vi "INTERFACE_HW_SW_FUERZA_PRENSIL_2009.vi"() -> ()   [LabVIEW 2009]
uses:
  <vilib>/Instr/_visa.llb/VISA Set IO Buffer Mask.ctl
  <vilib>/Instr/_visa.llb/VISA Configure Serial Port (Instr).vi
panel:
  out "GRAFICA DE LA FUERZA PRENSIL":cluster{dbl[], dbl[]}[](graph)
  out "F1":dbl format="%#_2g"
  out "F2":dbl format="%#_2g"
  out "F3":dbl format="%#_2g"
  in  "stop":bool
  out "Slide":u16(slide) scale=0.0..15.0
  out "Slide 2":u16(slide) scale=0.0..15.0
  out "Slide 3":u16(slide) scale=0.0..15.0
  out "Slide 4":u16(slide) scale=0.0..15.0
  out "Fprom":dbl format="%#_2g"
  out "F1 media":dbl format="%#.2g"
  out "F1 Max":dbl format="%#.2g"
  out "F2 media":dbl format="%#.2g"
  out "F2 Max":dbl format="%#.2g"
  out "F3 media":dbl format="%#.2g"
  out "F3 Max":dbl format="%#.2g"
  out "Fprom media":dbl format="%#.2g"
  out "Fprom Max":dbl format="%#.2g"
  out "Slide 5":u16(slide) scale=0.0..15.0 scale format="%.2f"
  out "F4":dbl format="%#_2g"
  out "F4 Max":dbl format="%#_2g"
  out "F4 Media":dbl format="%#_2g"
  out "No. de muestra":i32
  in  "MEDIR":bool
  out "Fprensil (N)":dbl
  out "Fprensil (kgf)":dbl
  in  "VISA resource name":refnum<visa-resource-name>
  # "L"
  # "i"
  # "V"
  # "INTERFASE PARA LA MEDICIÓN DE LA FUERZA PRENSIL"
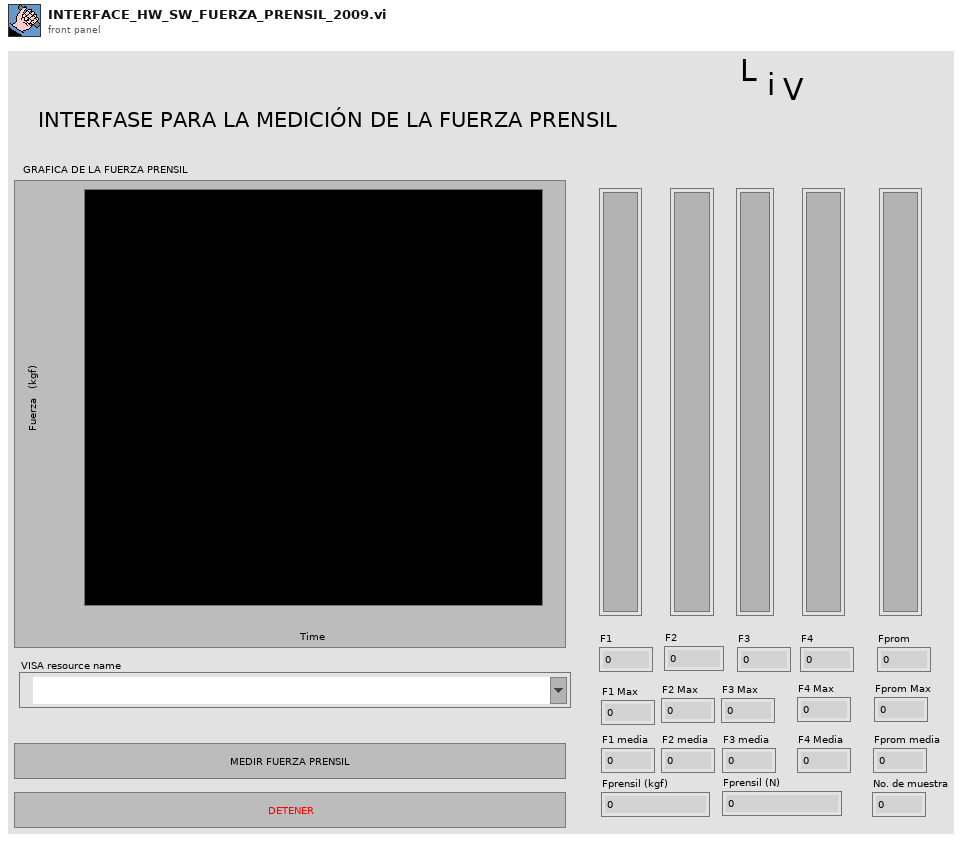
[diagram p1: front panel]
types:
  T1 = typedef "VISA Set IO Buffer Mask.ctl" = u16
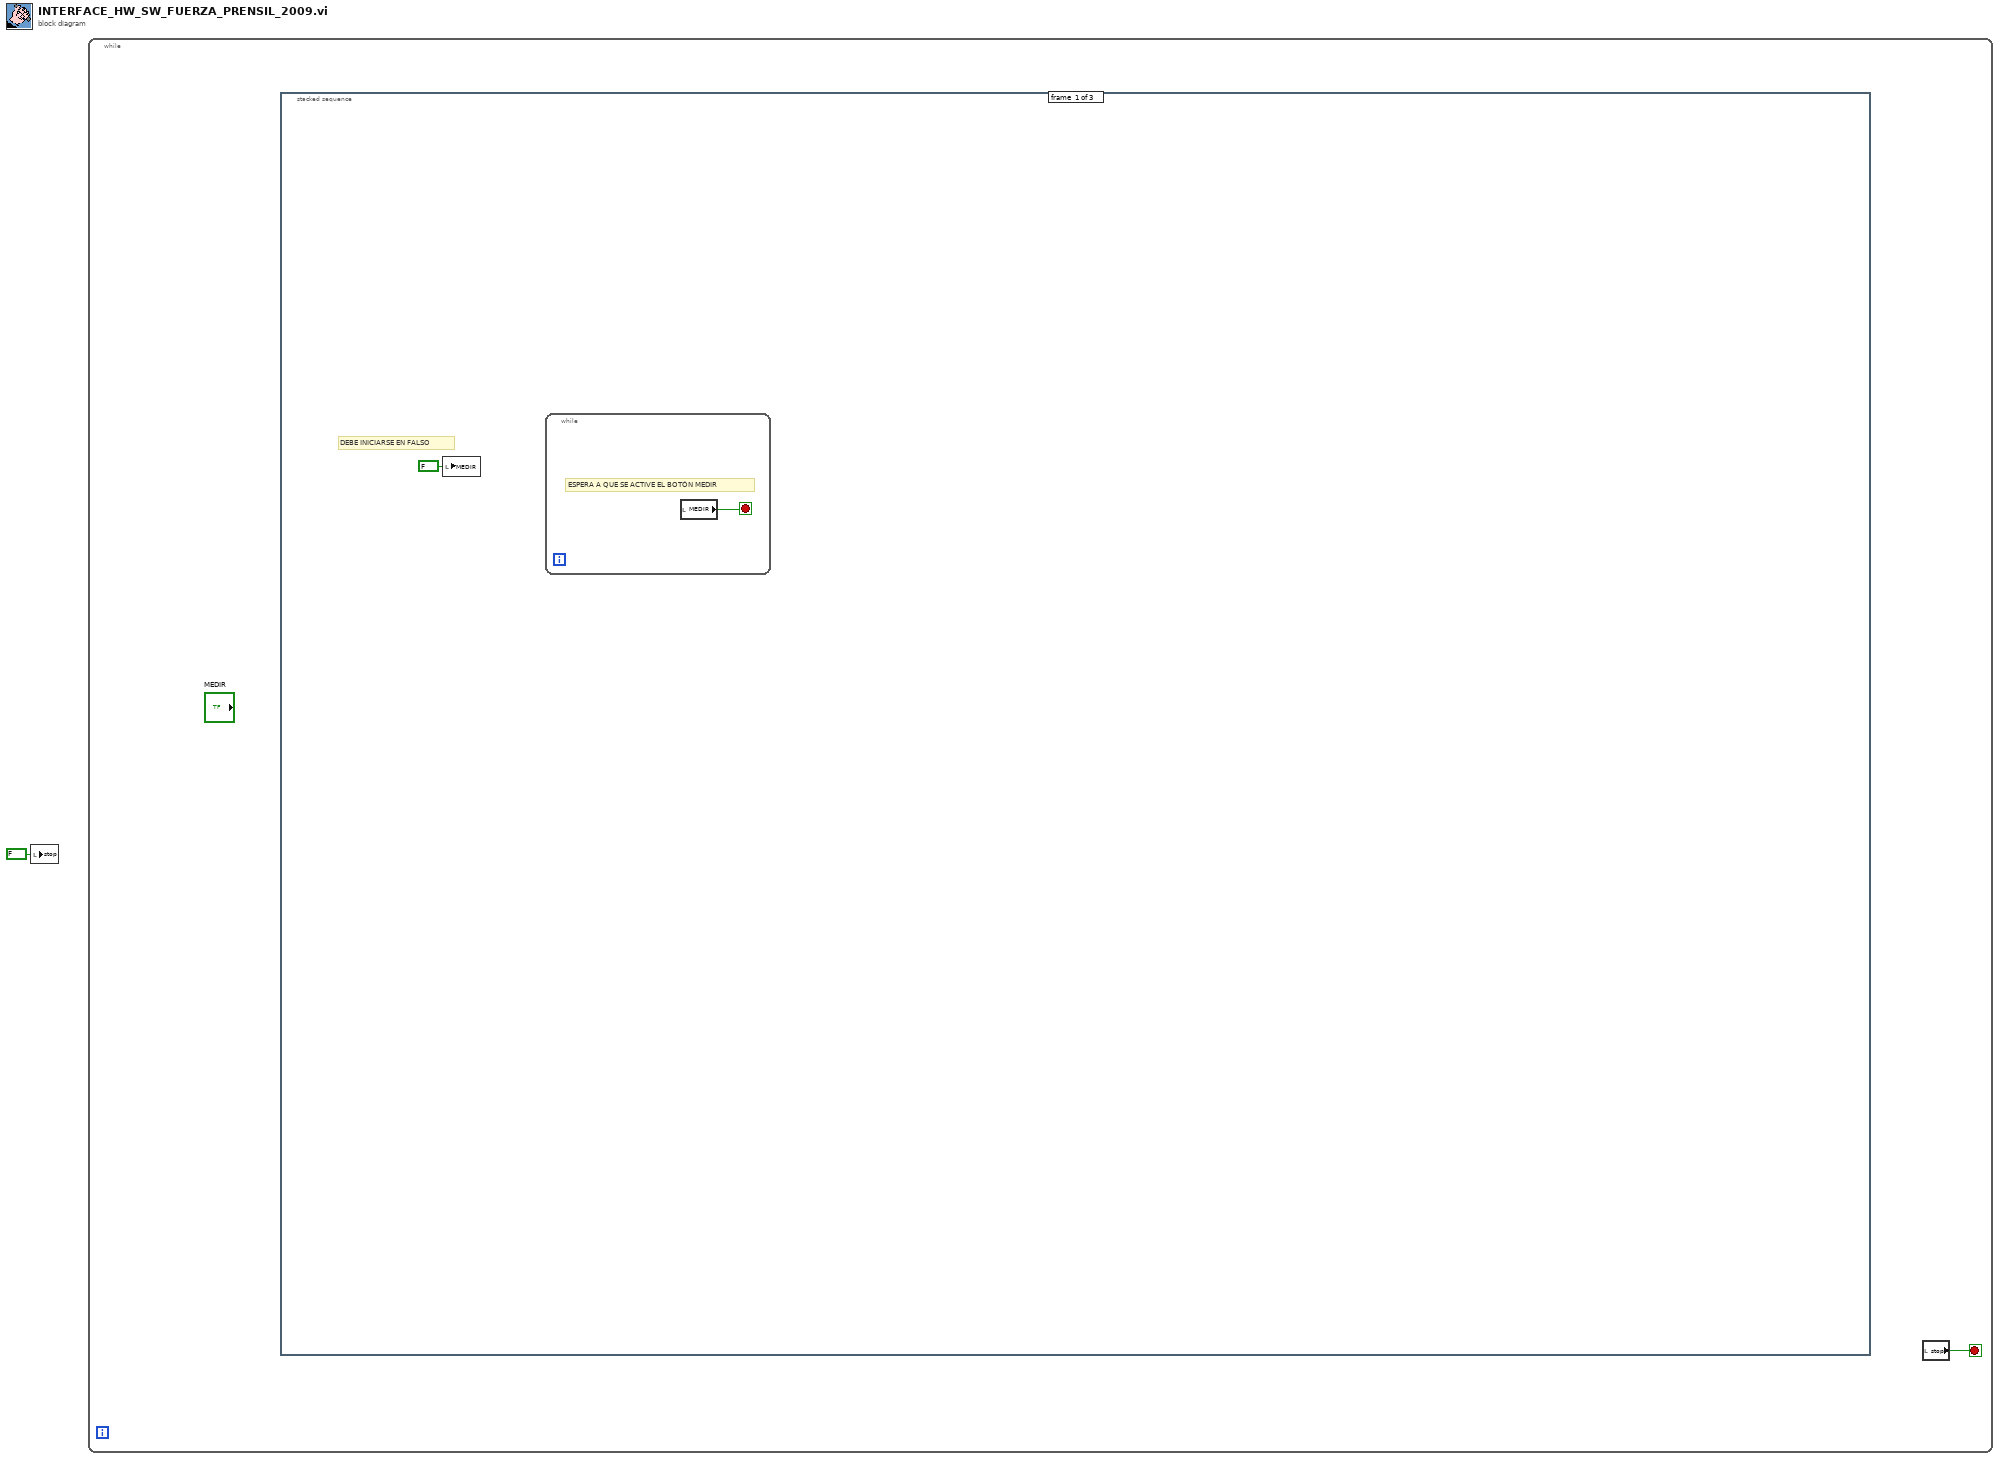
[diagram p0: block diagram]
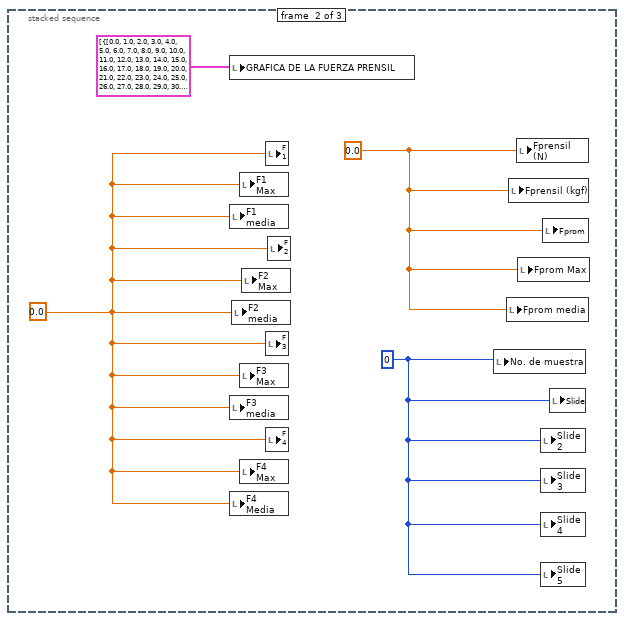
[diagram p2: hidden frame]
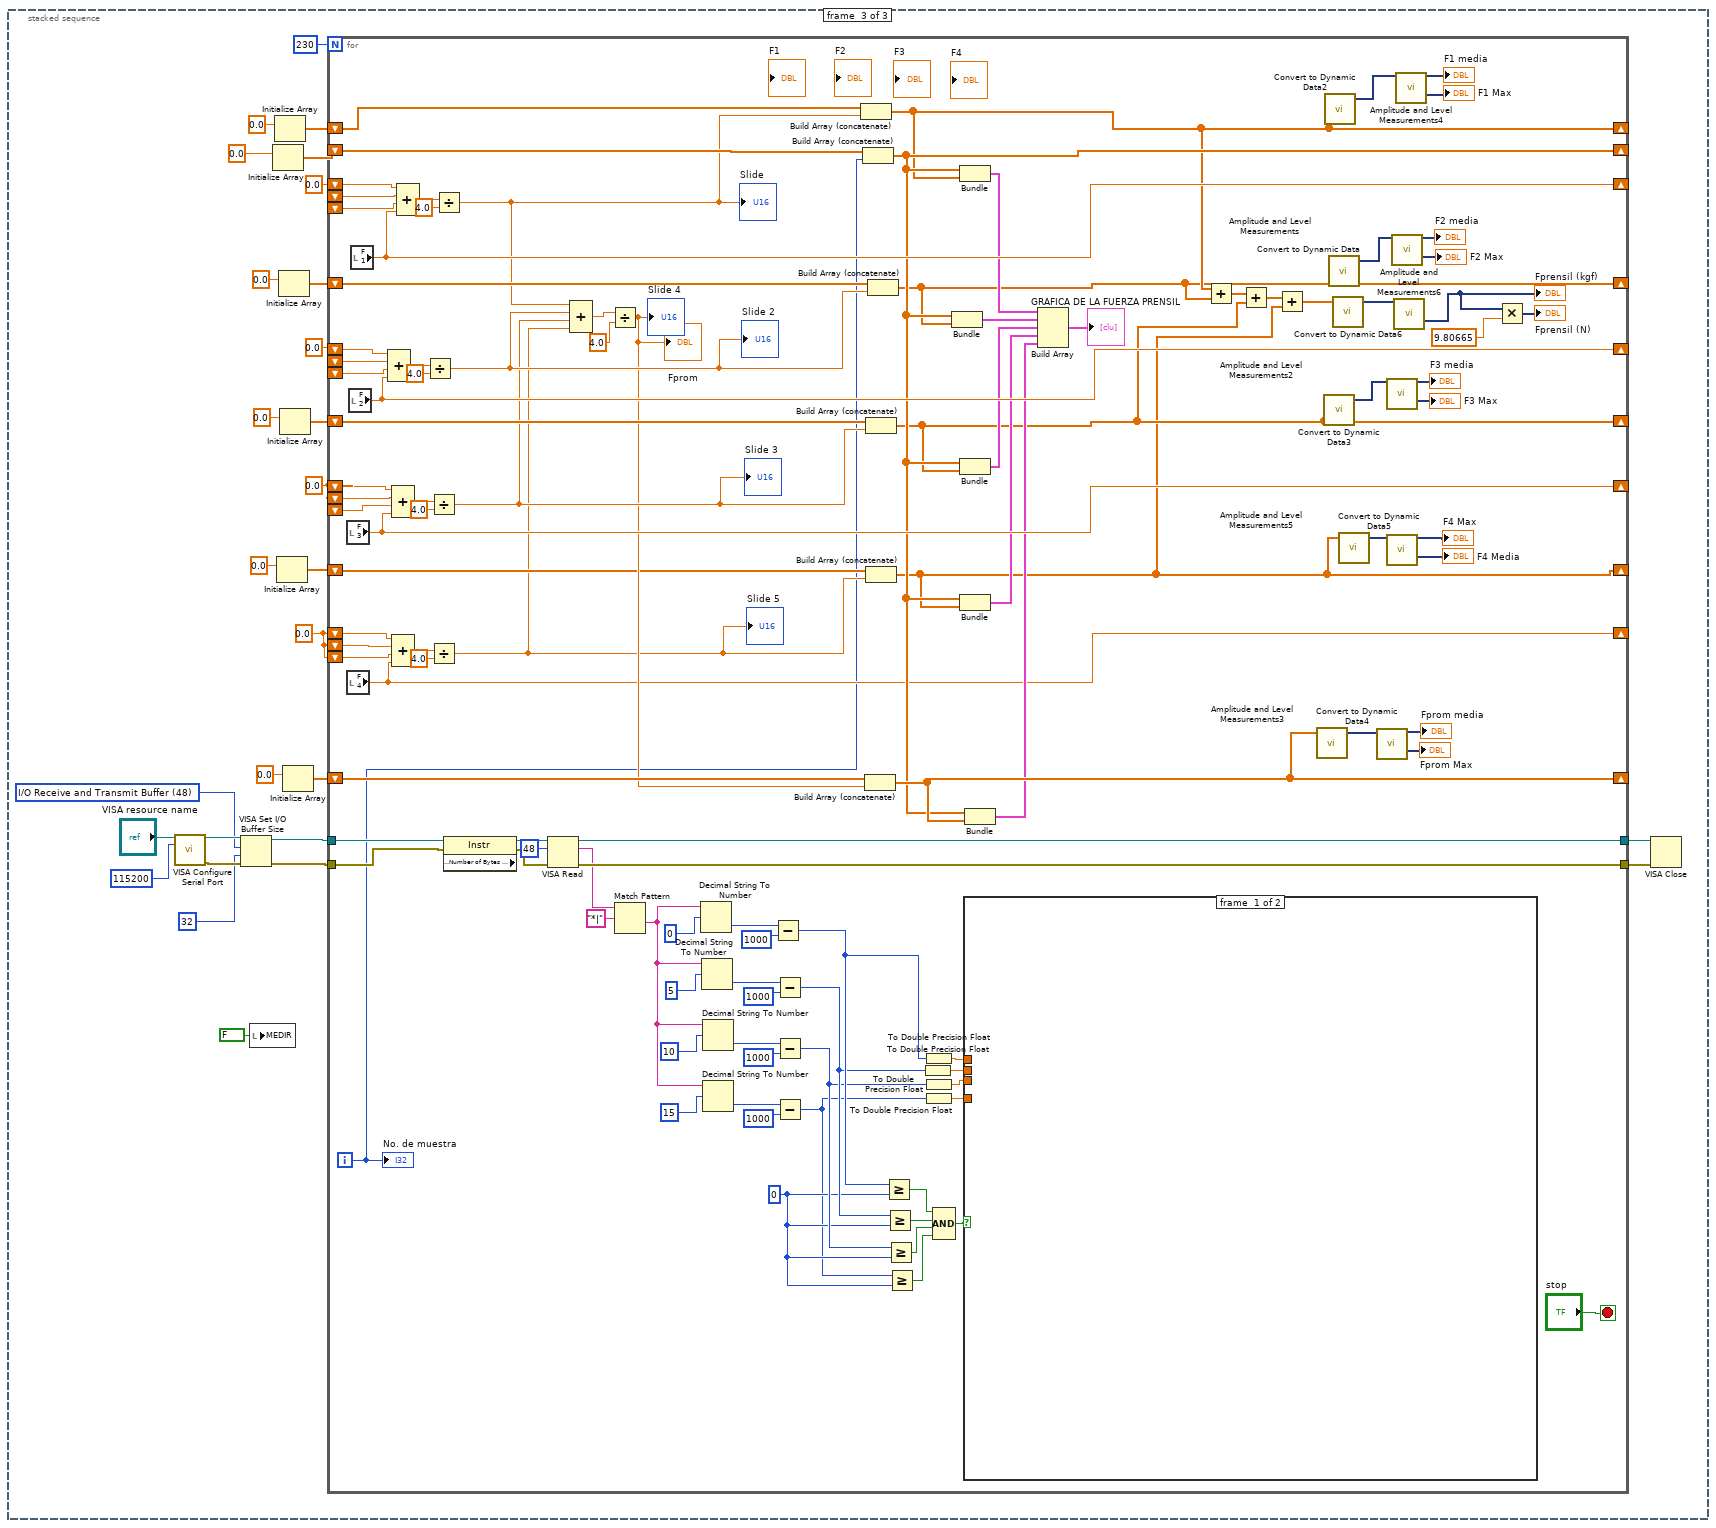
[diagram p3: hidden frame]
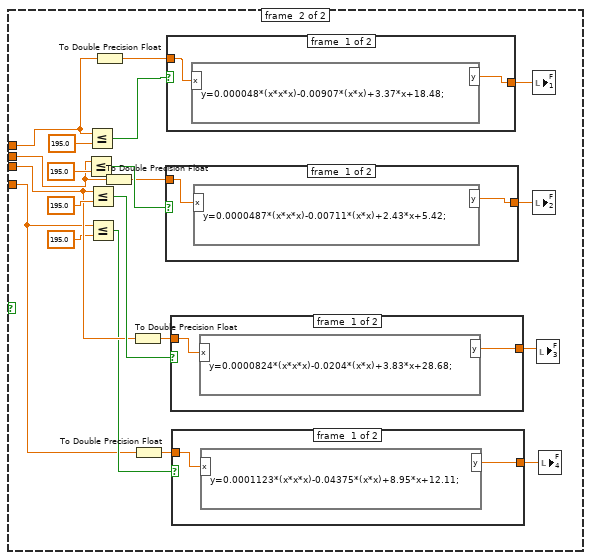
[diagram p4: hidden frame]
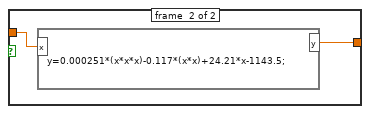
[diagram p5: hidden frame]
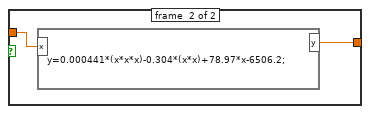
[diagram p6: hidden frame]
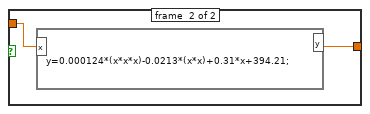
[diagram p7: hidden frame]
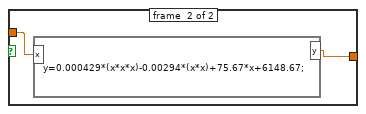
[diagram p8: hidden frame]
diagram:
  n1 = local write "stop"(FALSE ("stop")) -> ()
  n2 = while {
    stop <- w2 stop-if-true
    n3 = stacked-sequence {
      frame #0 {
        # "DEBE INICIARSE EN FALSO"
        n4 = local write "MEDIR"(FALSE ("MEDIR")) -> ()
        n5 = while {
          stop <- w4 stop-if-true
          # "ESPERA A QUE SE ACTIVE EL BOTÓN MEDIR"
          n6 = local read "MEDIR"() -> (w4:bool)
        }
      }
      frame #1 {
        w5 = 0.0 ("Fprensil (N)")
        w6 = 0.0 ("F1")
        w7 = 0 ("No. de muestra")
        n7 = local write "GRAFICA DE LA FUERZA PRENSIL"(cluster{dbl[], dbl[]}[] [{[0.0, 1.0, 2.0, 3.0, 4.0, 5.0, 6.0, 7.0, 8.0, 9.0, 10.0, 11.0, 12.0, 13.0, 14.0, 15.0, 16.0, 17.0, 18.0, 19.0, 20.0, 21.0, 22.0, 23.0, 24.0, 25.0, 26.0, 27.0, 28.0, 29.0, 30.0, 31.0, 32.0, 33.0, 34.0, 35.0, 36.0, 37.0, 38.0, 39.0, 40.0, 41.0, 42.0, 43.0, 44.0, 45.0, 46.0, 47.0, 48.0, 49.0, 50.0, 51.0, 52.0, 53.0, 54.0, 55.0, 56.0, 57.0, 58.0, 59.0, 60.0, 61.0, 62.0, 63.0, 64.0, 65.0, 66.0, 67.0, 68.0, 69.0, 70.0, 71.0, 72.0, 73.0, 74.0, 75.0, 76.0, 77.0, 78.0, 79.0, 80.0, 81.0, 82.0, 83.0, 84.0, 85.0, 86.0, 87.0, 88.0, 89.0, 90.0, 91.0, 92.0, 93.0, 94.0, 95.0, 96.0, 97.0, 98.0, 99.0, 100.0, 101.0, 102.0, 103.0, 104.0, 105.0, 106.0, 107.0, 108.0, 109.0, 110.0, 111.0, 112.0, 113.0, 114.0, 115.0, 116.0, 117.0, 118.0, 119.0, 120.0, 121.0, 122.0, 123.0, 124.0, 125.0, 126.0, 127.0, 128.0, 129.0, 130.0, 131.0, 132.0, 133.0, 134.0, 135.0, 136.0, 137.0, 138.0, 139.0, 140.0, 141.0, 142.0, 143.0, 144.0, 145.0, 146.0, 147.0, 148.0, 149.0, 150.0, 151.0, 152.0, 153.0, 154.0, 155.0, 156.0, 157.0, 158.0, 159.0, 160.0, 161.0, 162.0, 163.0, 164.0, 165.0, 166.0, 167.0, 168.0, 169.0, 170.0, 171.0, 172.0, 173.0, 174.0, 175.0, 176.0, 177.0, 178.0, 179.0, 180.0, 181.0, 182.0, 183.0, 184.0, 185.0, 186.0, 187.0, 188.0, 189.0, 190.0, 191.0, 192.0, 193.0, 194.0, 195.0, 196.0, 197.0, 198.0, 199.0, 200.0, 201.0, 202.0, 203.0, 204.0, 205.0, 206.0, 207.0, 208.0, 209.0, 210.0, 211.0, 212.0, 213.0, 214.0, 215.0, 216.0, 217.0, 218.0, 219.0, 220.0, 221.0, 222.0, 223.0, 224.0, 225.0, 226.0, 227.0, 228.0, 229.0], [0.0006720016874999999, 0.0013440033749999999, 0.0020160050625, 0.0026880067499999998, 0.0026880067499999998, 0.0026880067499999998, 0.0026880067499999998, 0.0026880067499999998, 0.0026880067499999998, 0.0026880067499999998, 0.0026880067499999998, 0.0026880067499999998, 0.0026880067499999998, 0.0026880067499999998, 0.0026880067499999998, 0.0026880067499999998, 0.0026880067499999998, 0.0026880067499999998, 0.0026880067499999998, 0.0026880067499999998, 0.0026880067499999998, 0.0026880067499999998, 0.0026880067499999998, 0.0026880067499999998, 0.0026880067499999998, 0.0026880067499999998, 0.0026880067499999998, 0.0026880067499999998, 0.0026880067499999998, 0.0026880067499999998, 0.0026880067499999998, 0.0026880067499999998, 0.0026880067499999998, 0.0026880067499999998, 0.0026880067499999998, 0.0026880067499999998, 0.0026880067499999998, 0.0026880067499999998, 0.0026880067499999998, 0.0026880067499999998, 0.0026880067499999998, 0.0026880067499999998, 0.0026880067499999998, 0.0026880067499999998, 0.0026880067499999998, 0.0026880067499999998, 0.0026880067499999998, 0.0026880067499999998, 0.0026880067499999998, 0.0026880067499999998, 0.0026880067499999998, 0.0026880067499999998, 0.0026880067499999998, 0.0026880067499999998, 0.0026880067499999998, 0.0026880067499999998, 0.0026880067499999998, 0.0026880067499999998, 0.0026880067499999998, 0.0026880067499999998, 0.0026880067499999998, 0.0026880067499999998, 0.0026880067499999998, 0.0026880067499999998, 0.0026880067499999998, 0.0026880067499999998, 0.0026880067499999998, 0.0026880067499999998, 0.0026880067499999998, 0.0026880067499999998, 0.0026880067499999998, 0.0026880067499999998, 0.0026880067499999998, 0.0026880067499999998, 0.0026880067499999998, 0.0026880067499999998, 0.0026880067499999998, 0.0026880067499999998, 0.0026880067499999998, 0.0026880067499999998, 0.0026880067499999998, 0.0026880067499999998, 0.0026880067499999998, 0.0026880067499999998, 0.0026880067499999998, 0.0026880067499999998, 0.0026880067499999998, 0.0026880067499999998, 0.0026880067499999998, 0.0026880067499999998, 0.0026880067499999998, 0.0026880067499999998, 0.0026880067499999998, 0.0026880067499999998, 0.0026880067499999998, 0.0026880067499999998, 0.0026880067499999998, 0.0026880067499999998, 0.0026880067499999998, 0.0026880067499999998, 0.0026880067499999998, 0.0026880067499999998, 0.0026880067499999998, 0.0026880067499999998, 0.0026880067499999998, 0.0026880067499999998, 0.0026880067499999998, 0.0026880067499999998, 0.0026880067499999998, 0.0026880067499999998, 0.0026880067499999998, 0.0026880067499999998, 0.0026880067499999998, 0.0026880067499999998, 0.0026880067499999998, 0.0026880067499999998, 0.0026880067499999998, 0.0026880067499999998, 0.0026880067499999998, 0.0026880067499999998, 0.0026880067499999998, 0.0026880067499999998, 0.0026880067499999998, 0.0026880067499999998, 0.0026880067499999998, 0.0026880067499999998, 0.0026880067499999998, 0.0026880067499999998, 0.0026880067499999998, 0.0026880067499999998, 0.0026880067499999998, 0.0026880067499999998, 0.0026880067499999998, 0.0026880067499999998, 0.0026880067499999998, 0.0026880067499999998, 0.0026880067499999998, 0.0026880067499999998, 0.0026880067499999998, 0.0026880067499999998, 0.0026880067499999998, 0.0026880067499999998, 0.0026880067499999998, 0.0026880067499999998, 0.0026880067499999998, 0.0026880067499999998, 0.0026880067499999998, 0.0026880067499999998, 0.0026880067499999998, 0.0026880067499999998, 0.0026880067499999998, 0.0026880067499999998, 0.0026880067499999998, 0.0026880067499999998, 0.0026880067499999998, 0.0026880067499999998, 0.0026880067499999998, 0.0026880067499999998, 0.0026880067499999998, 0.0026880067499999998, 0.0026880067499999998, 0.0026880067499999998, 0.0026880067499999998, 0.0026880067499999998, 0.0026880067499999998, 0.0026880067499999998, 0.0026880067499999998, 0.0026880067499999998, 0.0026880067499999998, 0.0026880067499999998, 0.0026880067499999998, 0.0026880067499999998, 0.0026880067499999998, 0.0026880067499999998, 0.0026880067499999998, 0.0026880067499999998, 0.0026880067499999998, 0.0026880067499999998, 0.0026880067499999998, 0.0026880067499999998, 0.0026880067499999998, 0.0026880067499999998, 0.0026880067499999998, 0.0026880067499999998, 0.0026880067499999998, 0.0026880067499999998, 0.0026880067499999998, 0.0026880067499999998, 0.0026880067499999998, 0.0026880067499999998, 0.0026880067499999998, 0.0026880067499999998, 0.0026880067499999998, 0.0026880067499999998, 0.0026880067499999998, 0.0026880067499999998, 0.0026880067499999998, 0.0026880067499999998, 0.0026880067499999998, 0.0026880067499999998, 0.0026880067499999998, 0.0026880067499999998, 0.0026880067499999998, 0.0026880067499999998, 0.0026880067499999998, 0.0026880067499999998, 0.0026880067499999998, 0.0026880067499999998, 0.0026880067499999998, 0.0026880067499999998, 0.0026880067499999998, 0.0026880067499999998, 0.0026880067499999998, 0.0026880067499999998, 0.0026880067499999998, 0.0026880067499999998, 0.0026880067499999998, 0.0026880067499999998, 0.0026880067499999998, 0.0026880067499999998, 0.0026880067499999998, 0.0026880067499999998, 0.0026880067499999998, 0.0026880067499999998, 0.0026880067499999998, 0.0026880067499999998, 0.0026880067499999998, 0.0026880067499999998, 0.0026880067499999998, 0.0026880067499999998]}, ...(5 in all)] ("GRAFICA DE LA FUERZA PRENSIL")) -> ()
        n8 = local write "F1 media"(w6) -> ()
        n9 = local write "F3 media"(w6) -> ()
        n10 = local write "F4 Media"(w6) -> ()
        n11 = local write "F2 media"(w6) -> ()
        n12 = local write "F1 Max"(w6) -> ()
        n13 = local write "F3 Max"(w6) -> ()
        n14 = local write "F4 Max"(w6) -> ()
        n15 = local write "F2 Max"(w6) -> ()
        n16 = local write "F1"(w6) -> ()
        n17 = local write "F3"(w6) -> ()
        n18 = local write "F4"(w6) -> ()
        n19 = local write "F2"(w6) -> ()
        n20 = local write "No. de muestra"(w7) -> ()
        n21 = local write "Fprom media"(w5) -> ()
        n22 = local write "Fprensil (kgf)"(w5) -> ()
        n23 = local write "Fprensil (N)"(w5) -> ()
        n24 = local write "Fprom Max"(w5) -> ()
        n25 = local write "Slide 2"(w7) -> ()
        n26 = local write "Slide 3"(w7) -> ()
        n27 = local write "Slide 4"(w7) -> ()
        n28 = local write "Slide 5"(w7) -> ()
        n29 = local write "Fprom"(w5) -> ()
        n30 = local write "Slide"(w7) -> ()
      }
      frame #2 {
        w14 = T1 48 items=["I/O Receive Buffer"=16, "I/O Transmit Buffer"=32, "I/O Receive and Transmit Buffer"=48] ("Mask")
        w20 = 0.0
        w29 = 0.0
        w30 = 0.0
        w34 = 0.0
        n31 = call-poly "VISA Configure Serial Port"("VISA resource name"="VISA resource name", "baud rate (9600)"=u32 115200) -> ("VISA resource name out"=w17:refnum<visa-resource-name>, "error out"=w18:errorcluster)  [unwired: 12 in]
        n32 = VISA Set I/O Buffer Size(VISA resource name=w17, mask (16)=w14, size (4096)=u32 32, error in (no error)=w18) -> (VISA resource name out=w12:refnum<visa-resource-name>, error out=w11:errorcluster)
        n33 = local write "MEDIR"(FALSE ("MEDIR")) -> ()
        n34 = Initialize Array(0.0 ("element")) -> (w31:dbl[])  [unwired: 1 in]
        n35 = Initialize Array(0.0 ("element")) -> (w32:dbl[])  [unwired: 1 in]
        n36 = Initialize Array(0.0 ("element")) -> (w21:dbl[])  [unwired: 1 in]
        n37 = Initialize Array(0.0 ("element")) -> (w26:dbl[])  [unwired: 1 in]
        n38 = Initialize Array(0.0 ("element")) -> (w25:dbl[])  [unwired: 1 in]
        n39 = Initialize Array(0.0 ("element")) -> (w23:dbl[])  [unwired: 1 in]
        n40 = for {
          N: 230 -> [_]
          tunnel: [w142] -> w10
          tunnel: [w141] -> w9
          tunnel: w12 -> [w130]
          tunnel: w11 -> [w129]
          shift-right: [w105] -> _
          shift-left: w34 -> [w124]
          shift-left: w34 -> [w123]
          shift-left: w34 -> [w122]
          shift-right: [w45] -> _
          shift-left: w32 -> [w119]
          shift-right: [w64] -> _
          shift-left: w31 -> [w118]
          shift-right: [w104] -> _
          shift-left: w30 -> [w115]
          shift-left: w30 -> [w114]
          shift-left: w30 -> [w113]
          shift-right: [w103] -> _
          shift-left: w29 -> [w110]
          shift-left: w29 -> [w109]
          shift-left: w29 -> [w108]
          shift-right: [w44] -> _
          shift-left: w26 -> [w107]
          shift-right: [w43] -> _
          shift-left: w25 -> [w106]
          shift-right: [w80] -> _
          shift-left: w23 -> [w91]
          shift-right: [w42] -> _
          shift-left: w21 -> [w70]
          shift-right: [w59] -> _
          shift-left: w20 -> [w67]
          shift-left: w20 -> [w66]
          shift-left: w20 -> [w65]
          i -> [w49]
          stop <- "stop" stop-if-true
          w56 = 0 ("y")
          n41 = local read "F3"() -> (w103:dbl)
          n42 = local read "F4"() -> (w59:dbl)
          n43 = local read "F2"() -> (w104:dbl)
          n44 = local read "F1"() -> (w105:dbl)
          n45 = Compound Arithmetic op=ADD(w115, w114, w113, w104) -> (w117:dbl)
          n46 = Compound Arithmetic op=ADD(w110, w109, w108, w103) -> (w112:dbl)
          n47 = Compound Arithmetic op=ADD(w67, w66, w65, w59) -> (w69:dbl)
          n48 = Compound Arithmetic op=ADD(w124, w123, w122, w105) -> (w121:dbl)
          n49 = Divide(x=w117, y=4.0) -> (x/y=w95:dbl)
          "Slide 2" <- w95
          n50 = Divide(x=w112, y=4.0) -> (x/y=w94:dbl)
          "Slide 3" <- w94
          n51 = Divide(x=w69, y=4.0) -> (x/y=w51:dbl)
          "Slide 5" <- w51
          n52 = Divide(x=w121, y=4.0) -> (x/y=w96:dbl)
          "Slide" <- w96
          n53 = property class="Instr" props=["Serial Settings:Number of Bytes at Serial Port"](reference=w130, error in=w129) -> (reference out=w145:refnum<visa-resource-name>, error out=w144:errorcluster)  [unwired: 1 out]
          n54 = VISA Read(VISA resource name=w145, byte count=u32 48, error in (no error)=w144) -> (VISA resource name out=w142:refnum<visa-resource-name>, read buffer=w131:string, error out=w141:errorcluster)  [unwired: 1 out]
          n55 = Compound Arithmetic op=ADD(w96, w95, w94, w51) -> (w93:dbl)
          n56 = Divide(x=w93, y=4.0) -> (x/y=w90:dbl)
          "Slide 4" <- w90
          "Fprom" <- w90
          n57 = Match Pattern(string=w131, regular expression="*|") -> (after substring=w52:string)  [unwired: 1 in, 3 out]
          n58 = Decimal String To Number(string=w52, offset=0) -> (number=w137:i32)  [unwired: 1 in, 1 out]
          n59 = Decimal String To Number(string=w52, offset=5) -> (number=w133:i32)  [unwired: 1 in, 1 out]
          n60 = Decimal String To Number(string=w52, offset=10) -> (number=w132:i32)  [unwired: 1 in, 1 out]
          n61 = Decimal String To Number(string=w52, offset=15) -> (number=w53:i32)  [unwired: 1 in, 1 out]
          n62 = Subtract(x=w137, y=1000) -> (x-y=w89:i32)
          n63 = Subtract(x=w133, y=1000) -> (x-y=w87:i32)
          n64 = Subtract(x=w132, y=1000) -> (x-y=w85:i32)
          n65 = Subtract(x=w53, y=1000) -> (x-y=w48:i32)
          n66 = Build Array (concatenate)(w119, w96) -> (w45:dbl[])
          n67 = Build Array (concatenate)(w118, w49) -> (w64:dbl[])
          n68 = Build Array (concatenate)(w91, w90) -> (w80:dbl[])
          n69 = Build Array (concatenate)(w106, w94) -> (w43:dbl[])
          n70 = Build Array (concatenate)(w70, w51) -> (w42:dbl[])
          n71 = Build Array (concatenate)(w107, w95) -> (w44:dbl[])
          n72 = Greater Or Equal?(x=w89, y=w56) -> (x >= y?=w127:bool)
          n73 = Greater Or Equal?(x=w87, y=w56) -> (x >= y?=w128:bool)
          n74 = Greater Or Equal?(x=w85, y=w56) -> (x >= y?=w126:bool)
          n75 = Greater Or Equal?(x=w48, y=w56) -> (x >= y?=w57:bool)
          n76 = To Double Precision Float(number=w87) -> (double precision float=w86:dbl)
          n77 = To Double Precision Float(number=w89) -> (double precision float=w88:dbl)
          n78 = To Double Precision Float(number=w85) -> (double precision float=w84:dbl)
          n79 = To Double Precision Float(number=w48) -> (double precision float=w58:dbl)
          n80 = Compound Arithmetic op=AND(w127, w128, w126, w57) -> (w125:bool)
          n81 = Bundle(w64, w44) -> (w101:cluster{dbl[], dbl[]})  [unwired: 1 in]
          n82 = Bundle(w64, w45) -> (w102:cluster{dbl[], dbl[]})  [unwired: 1 in]
          n83 = Bundle(w64, w43) -> (w100:cluster{dbl[], dbl[]})  [unwired: 1 in]
          n84 = Bundle(w64, w42) -> (w62:cluster{dbl[], dbl[]})  [unwired: 1 in]
          n85 = case shown="True" w125 {
            tunnel: w88 -> [_ w159]
            tunnel: w86 -> [_ w154]
            tunnel: w84 -> [_ w157]
            tunnel: w58 -> [_ w146]
            frame #0 {
            }
            frame #1 {
              n86 = Less Or Equal?(x=w154, y=195.0) -> (x <= y?=w161:bool)
              n87 = Less Or Equal?(x=w159, y=195.0) -> (x <= y?=w162:bool)
              n88 = Less Or Equal?(x=w157, y=195.0) -> (x <= y?=w160:bool)
              n89 = Less Or Equal?(x=w146, y=195.0) -> (x <= y?=w147:bool)
              n90 = To Double Precision Float(number=w159) -> (double precision float=w158:dbl)
              n91 = To Double Precision Float(number=w154) -> (double precision float=w155:dbl)
              n92 = To Double Precision Float(number=w157) -> (double precision float=w156:dbl)
              n93 = To Double Precision Float(number=w146) -> (double precision float=w150:dbl)
              n94 = case shown="False" w161 {
                tunnel: w155 -> [w175 w177]
                tunnel: [w174 w176] -> w152
                frame #0 {
                  n95 = formula code="y=0.0000487*(x*x*x)-0.00711*(x*x)+2.43*x+5.42;"("x"=w175) -> ("y"=w174:dbl)
                }
                frame #1 {
                  n96 = formula code="y=0.000124*(x*x*x)-0.0213*(x*x)+0.31*x+394.21;"("x"=w177) -> ("y"=w176:dbl)
                }
              }
              n97 = case shown="False" w162 {
                tunnel: w158 -> [w179 w181]
                tunnel: [w178 w180] -> w153
                frame #0 {
                  n98 = formula code="y=0.000048*(x*x*x)-0.00907*(x*x)+3.37*x+18.48;"("x"=w179) -> ("y"=w178:dbl)
                }
                frame #1 {
                  n99 = formula code="y=0.000429*(x*x*x)-0.00294*(x*x)+75.67*x+6148.67;"("x"=w181) -> ("y"=w180:dbl)
                }
              }
              n100 = case shown="False" w160 {
                tunnel: w156 -> [w171 w173]
                tunnel: [w170 w172] -> w151
                frame #0 {
                  n101 = formula code="y=0.0000824*(x*x*x)-0.0204*(x*x)+3.83*x+28.68;"("x"=w171) -> ("y"=w170:dbl)
                }
                frame #1 {
                  n102 = formula code="y=0.000441*(x*x*x)-0.304*(x*x)+78.97*x-6506.2;"("x"=w173) -> ("y"=w172:dbl)
                }
              }
              n103 = case shown="False" w147 {
                tunnel: w150 -> [w167 w169]
                tunnel: [w166 w168] -> w149
                frame #0 {
                  n104 = formula code="y=0.0001123*(x*x*x)-0.04375*(x*x)+8.95*x+12.11;"("x"=w167) -> ("y"=w166:dbl)
                }
                frame #1 {
                  n105 = formula code="y=0.000251*(x*x*x)-0.117*(x*x)+24.21*x-1143.5;"("x"=w169) -> ("y"=w168:dbl)
                }
              }
              n106 = local write "F1"(w153) -> ()
              n107 = local write "F2"(w152) -> ()
              n108 = local write "F3"(w151) -> ()
              n109 = local write "F4"(w149) -> ()
            }
          }
          n110 = Bundle(w64, w80) -> (w63:cluster{dbl[], dbl[]})  [unwired: 1 in]
          n111 = Build Array(w102, w101, w100, w62, w63) -> (→"GRAFICA DE LA FUERZA PRENSIL":cluster{dbl[], dbl[]}[])
          n112 = Add(x=w45, y=w44) -> (x+y=w47:dbl[])
          n113 = Add(x=w47, y=w43) -> (x+y=w46:dbl[])
          n114 = Add(x=w46, y=w42) -> (x+y=w40:dbl[])
          n115 = call "Convert to Dynamic Data4"("Array"=w80) -> ("Dynamic Data Type"=w79:dynamicdata)  [unwired: 3 in]
          n116 = call "Convert to Dynamic Data3"("Array"=w43) -> ("Dynamic Data Type"=w81:dynamicdata)  [unwired: 3 in]
          n117 = call "Convert to Dynamic Data2"("Array"=w45) -> ("Dynamic Data Type"=w82:dynamicdata)  [unwired: 3 in]
          n118 = call "Convert to Dynamic Data"("Array"=w44) -> ("Dynamic Data Type"=w83:dynamicdata)  [unwired: 3 in]
          n119 = call "Convert to Dynamic Data6"("Array"=w40) -> ("Dynamic Data Type"=w41:dynamicdata)  [unwired: 3 in]
          n120 = call "Convert to Dynamic Data5"("Array"=w42) -> ("Dynamic Data Type"=w61:dynamicdata)  [unwired: 3 in]
          n121 = call "Amplitude and Level Measurements3"("Signals"=w79) -> ("Mean (DC)"=→"Fprom media":dynamicdata, "Positive Peak"=→"Fprom Max":dynamicdata)  [unwired: 12 in, 1 out]
          n122 = call "Amplitude and Level Measurements2"("Signals"=w81) -> ("Mean (DC)"=→"F3 media":dynamicdata, "Positive Peak"=→"F3 Max":dynamicdata)  [unwired: 12 in, 1 out]
          n123 = call "Amplitude and Level Measurements5"("Signals"=w61) -> ("Mean (DC)"=→"F4 Max":dynamicdata, "Positive Peak"=→"F4 Media":dynamicdata)  [unwired: 12 in, 1 out]
          n124 = call "Amplitude and Level Measurements"("Signals"=w83) -> ("Mean (DC)"=→"F2 media":dynamicdata, "Positive Peak"=→"F2 Max":dynamicdata)  [unwired: 12 in, 1 out]
          n125 = call "Amplitude and Level Measurements6"("Signals"=w41) -> ("Positive Peak"=w37:dynamicdata)  [unwired: 12 in, 2 out]
          "Fprensil (kgf)" <- w37
          n126 = call "Amplitude and Level Measurements4"("Signals"=w82) -> ("Mean (DC)"=→"F1 media":dynamicdata, "Positive Peak"=→"F1 Max":dynamicdata)  [unwired: 12 in, 1 out]
          n127 = Multiply(x=w37, y=9.80665) -> (x*y=→"Fprensil (N)":dynamicdata)
          "No. de muestra" <- w49
        }
        n128 = VISA Close(VISA resource name=w10, error in (no error)=w9) -> ()  [unwired: 1 out]
      }
    }
    n129 = local read "stop"() -> (w2:bool)
  }
